vi "Intersperse Data with Invalid Data  2 parallel samples(3 channel).vi"(1 "Intersperse Ratio":dbl=0.1, 5 "Channel0 Input":dbl[](array[numeric]) format="%.16g", 7 "Channel1 Input":dbl[](array[numeric]) format="%.16g", 9 "Channel2 Input":dbl[](array[numeric]) format="%.16g") -> (6 "Channel0 Output":dbl[](array[numeric]), 8 "Channel1 Output":dbl[](array[numeric]), 10 "Channel2 Output":dbl[](array[numeric]), 15 "Data Valid":bool[](array[boolean]))   [LabVIEW 2011]
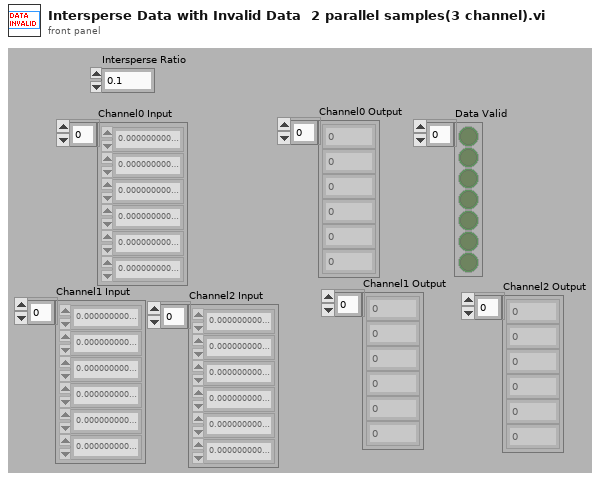
[diagram p1: front panel]
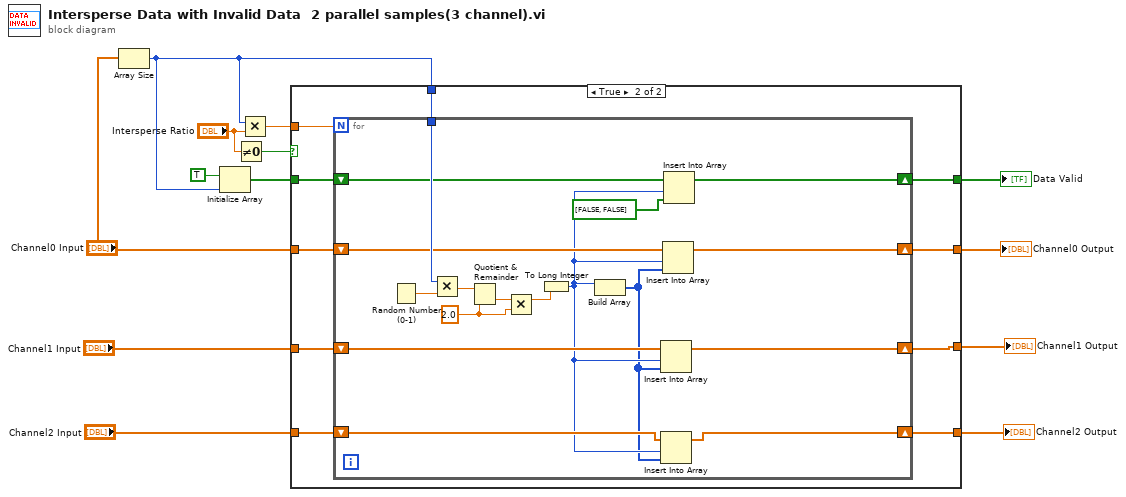
[diagram p0: block diagram]
diagram:
  n1 = Array Size(array="Channel0 Input") -> (size(s)=w12:i32)
  n2 = Initialize Array(TRUE, w12) -> (w10:bool[])
  n3 = Not Equal To 0?(x="Intersperse Ratio") -> (x != 0?=w3:bool)
  n4 = Multiply(x=w12, y="Intersperse Ratio") -> (x*y=w5:dbl)
  n5 = case shown="True" w3 {
    tunnel: "Channel0 Input" -> [w17 w27]
    tunnel: w12 -> [_ w26]
    tunnel: w10 -> [w16 w25]
    tunnel: [w16 w24] -> w9
    tunnel: [w17 w23] -> w8
    tunnel: "Channel1 Input" -> [w15 w22]
    tunnel: [w15 w21] -> w6
    tunnel: w5 -> [_ w20]
    tunnel: "Channel2 Input" -> [w14 w19]
    tunnel: [w14 w18] -> w1
    frame False {
    }
    frame True {
      n6 = for {
        N: w20 -> [_]
        tunnel: w26 -> [w44]
        shift-right: [w38] -> w23
        shift-left: w27 -> [w43]
        shift-right: [w39] -> w24
        shift-left: w25 -> [w42]
        shift-right: [w37] -> w21
        shift-left: w22 -> [w41]
        shift-right: [w36] -> w18
        shift-left: w19 -> [w40]
        w28 = 2.0 ("y")
        n7 = Random Number (0-1)() -> (number: 0 to 1=w35:dbl)
        n8 = Multiply(x=w44, y=w35) -> (x*y=w31:dbl)
        n9 = Quotient & Remainder(x=w31, y=w28) -> (floor(x/y)=w30:dbl)  [unwired: 1 out]
        n10 = Multiply(x=w30, y=w28) -> (x*y=w29:dbl)
        n11 = To Long Integer(number=w29) -> (32bit integer=w33:i32)
        n12 = Build Array(w33, w33) -> (w32:i32[])
        n13 = Insert Into Array(array=w41, index=w33, new element=w32) -> (w37:dbl[])
        n14 = Insert Into Array(array=w40, index=w33, new element=w32) -> (w36:dbl[])
        n15 = Insert Into Array(array=w43, index=w33, new element=w32) -> (w38:dbl[])
        n16 = Insert Into Array(array=w42, index=w33, new element=bool[] [FALSE, FALSE]) -> (w39:bool[])
      }
    }
  }
  "Data Valid" <- w9
  "Channel0 Output" <- w8
  "Channel1 Output" <- w6
  "Channel2 Output" <- w1
